vi "EncoderInit.vi"(8 "error in (no error)":errorcluster, 10 "Pin":u8, 11 "AdaFruit-Seesaw in":refnum<class "AdaFruit-Seesaw.lvclass">) -> (0 "error out":errorcluster, 3 "AdaFruit-Seesaw out":refnum<class "AdaFruit-Seesaw.lvclass">)   [LabVIEW 2020, in "CTI-Peripheral.lvlib" / "AdaFruit-Seesaw.lvclass"]
uses:
  AdaFruit-Seesaw.lvclass
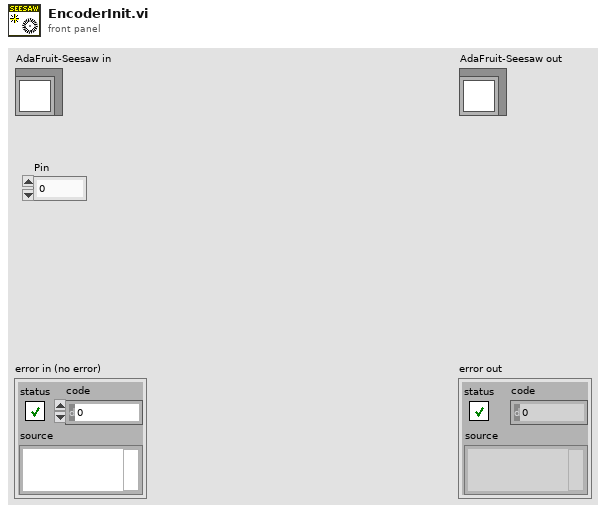
[diagram p1: front panel]
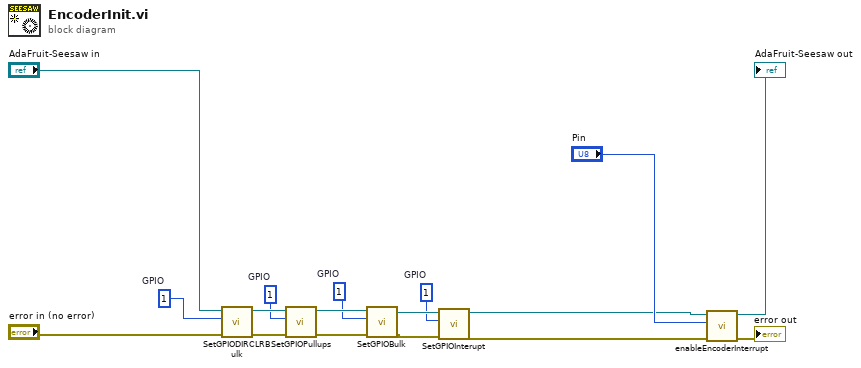
[diagram p0: block diagram]
diagram:
  w4 = u32 1  # GPIO
  w6 = u32 1  # GPIO
  w9 = u32 1  # GPIO
  w12 = u32 1  # GPIO
  n1 = call "SetGPIODIRCLRBulk.vi"("error in (no error)"="error in (no error)", "GPIO"=w12, "AdaFruit-Seesaw in"="AdaFruit-Seesaw in") -> ("error out"=w10:errorcluster, "AdaFruit-Seesaw out"=w11:refnum<class "AdaFruit-Seesaw.lvclass">)  [unwired: 7 in]
  n2 = call "SetGPIOPullups.vi"("error in (no error)"=w10, "GPIO"=w9, "AdaFruit-Seesaw in"=w11) -> ("error out"=w8:errorcluster, "AdaFruit-Seesaw out"=w7:refnum<class "AdaFruit-Seesaw.lvclass">)  [unwired: 7 in]
  n3 = call "SetGPIOBulk.vi"("error in (no error)"=w8, "GPIO"=w6, "AdaFruit-Seesaw in"=w7) -> ("error out"=w3:errorcluster, "AdaFruit-Seesaw out"=w5:refnum<class "AdaFruit-Seesaw.lvclass">)  [unwired: 7 in]
  n4 = call "SetGPIOInterupt.vi"("error in (no error)"=w3, "GPIO"=w4, "AdaFruit-Seesaw in"=w5) -> ("error out"=w2:errorcluster, "AdaFruit-Seesaw out"=w1:refnum<class "AdaFruit-Seesaw.lvclass">)  [unwired: 7 in]
  n5 = call "enableEncoderInterrupt.vi"("error in (no error)"=w2, "Encoder"="Pin", "AdaFruit-Seesaw in"=w1) -> ("error out"=→"error out":errorcluster, "AdaFruit-Seesaw out"=→"AdaFruit-Seesaw out":refnum<class "AdaFruit-Seesaw.lvclass">)  [unwired: 7 in]
